vi "svx_Colormap Calculate Order Frequency from Cursor.vi"(9 "CursLoc":cluster{"X":dbl, "Y":dbl}, 10 "plot type":T1(ring), 11 "speed profile":cluster{"time [s]":dbl[], "speed [rpm]":dbl[]}) -> (2 "Order type":dbl[](array[numeric])=[10.0], 3 "Frequency type":dbl[](array[numeric])=[10.0])   [LabVIEW 2017, in "SVX Colormap.xctl"]
uses:
  <vilib>/addons/_XControls/Colormap/SVX Colormap.xctl
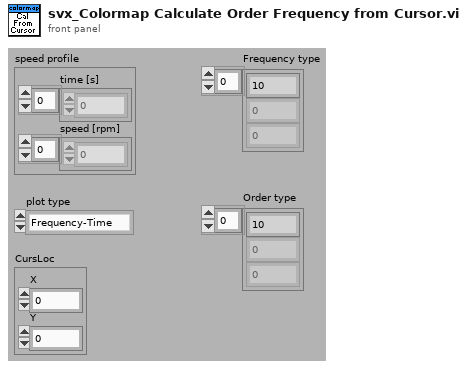
[diagram p1: front panel]
types:
  T1 = enum16{"Frequency-Time", "Time-Frequency", "Order-Time", "Time-Order", "Frequency-RPM", "RPM-Frequency", "Order-RPM", "RPM-Order"}
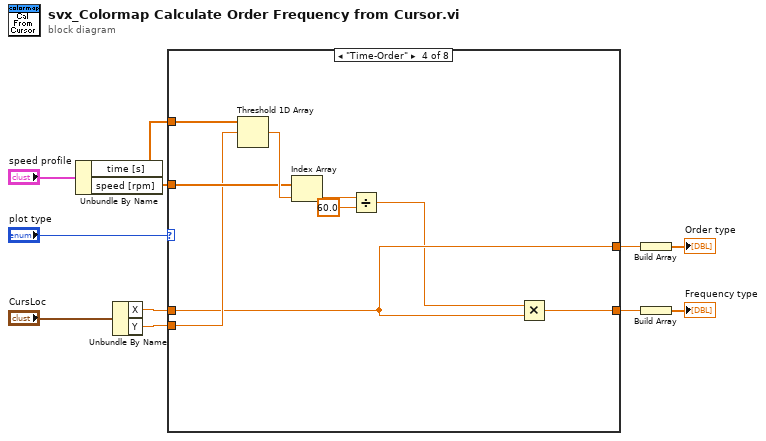
[diagram p0: block diagram]
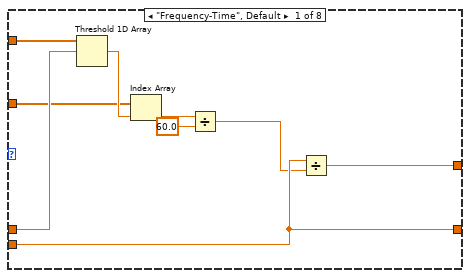
[diagram p2: hidden frame]
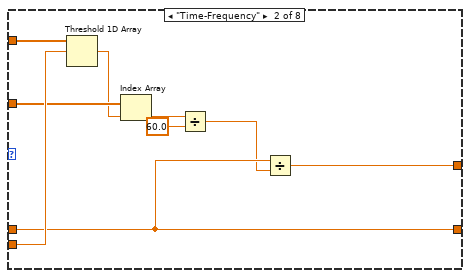
[diagram p3: hidden frame]
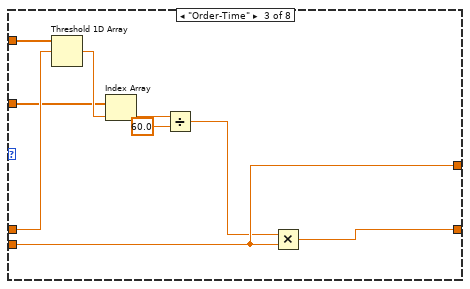
[diagram p4: hidden frame]
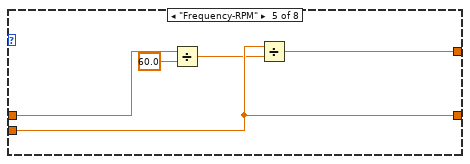
[diagram p5: hidden frame]
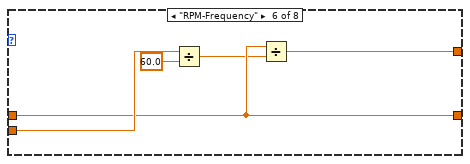
[diagram p6: hidden frame]
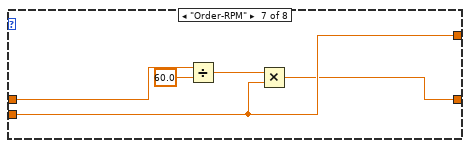
[diagram p7: hidden frame]
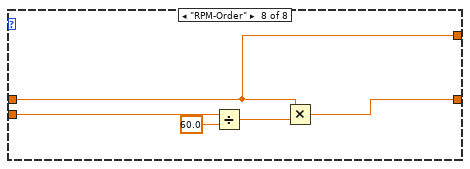
[diagram p8: hidden frame]
diagram:
  n1 = Unbundle By Name("speed profile") -> ("time [s]"=w8:dbl[], "speed [rpm]"=w6:dbl[])
  n2 = Unbundle By Name("CursLoc") -> ("X"=w5:dbl, "Y"=w7:dbl)
  n3 = case shown="\"Time-Order\"" "plot type" {
    tunnel: w8 -> [w17 w29 w35 w45 _ _ _ _]
    tunnel: w7 -> [w13 w28 w32 w41 w49 w56 w60 w66]
    tunnel: w6 -> [w15 w27 w33 w44 _ _ _ _]
    tunnel: [w13 w25 w31 w42 w49 w55 w59 w65] -> w4
    tunnel: w5 -> [w16 w25 w34 w40 w51 w55 w61 w64]
    tunnel: [w14 w22 w32 w40 w50 w54 w60 w64] -> w2
    frame "Frequency-Time", Default {
      n4 = Threshold 1D Array(2:w16, 3:w17) -> (0:w20:dbl)  [unwired: 1 in]
      n5 = Index Array(array=w15, index=w20) -> (element=w19:dbl)
      n6 = Divide(x=w19, y=60.0) -> (x/y=w12:dbl)
      n7 = Divide(x=w13, y=w12) -> (x/y=w14:dbl)
    }
    frame "Time-Frequency" {
      n8 = Threshold 1D Array(2:w28, 3:w29) -> (0:w26:dbl)  [unwired: 1 in]
      n9 = Index Array(array=w27, index=w26) -> (element=w24:dbl)
      n10 = Divide(x=w24, y=60.0) -> (x/y=w21:dbl)
      n11 = Divide(x=w25, y=w21) -> (x/y=w22:dbl)
    }
    frame "Order-Time" {
      n12 = Threshold 1D Array(2:w34, 3:w35) -> (0:w38:dbl)  [unwired: 1 in]
      n13 = Index Array(array=w33, index=w38) -> (element=w37:dbl)
      n14 = Divide(x=w37, y=60.0) -> (x/y=w30:dbl)
      n15 = Multiply(x=w30, y=w32) -> (x*y=w31:dbl)
    }
    frame "Time-Order" {
      n16 = Threshold 1D Array(2:w41, 3:w45) -> (0:w47:dbl)  [unwired: 1 in]
      n17 = Index Array(array=w44, index=w47) -> (element=w43:dbl)
      n18 = Divide(x=w43, y=60.0) -> (x/y=w39:dbl)
      n19 = Multiply(x=w39, y=w40) -> (x*y=w42:dbl)
    }
    frame "Frequency-RPM" {
      n20 = Divide(x=w51, y=60.0) -> (x/y=w48:dbl)
      n21 = Divide(x=w49, y=w48) -> (x/y=w50:dbl)
    }
    frame "RPM-Frequency" {
      n22 = Divide(x=w56, y=60.0) -> (x/y=w53:dbl)
      n23 = Divide(x=w55, y=w53) -> (x/y=w54:dbl)
    }
    frame "Order-RPM" {
      n24 = Divide(x=w61, y=60.0) -> (x/y=w58:dbl)
      n25 = Multiply(x=w58, y=w60) -> (x*y=w59:dbl)
    }
    frame "RPM-Order" {
      n26 = Divide(x=w66, y=60.0) -> (x/y=w63:dbl)
      n27 = Multiply(x=w64, y=w63) -> (x*y=w65:dbl)
    }
  }
  n28 = Build Array(w2) -> (→"Order type":dbl[])
  n29 = Build Array(w4) -> (→"Frequency type":dbl[])
